vi "ExpressVIElapsedTime.vi"() -> ()   [LabVIEW 2019]
panel:
  in  "stop":bool
  in  "Time Target (s)":dbl=5.0
  out "Boolean":bool
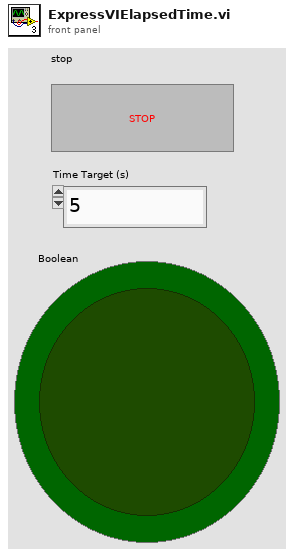
[diagram p1: front panel]
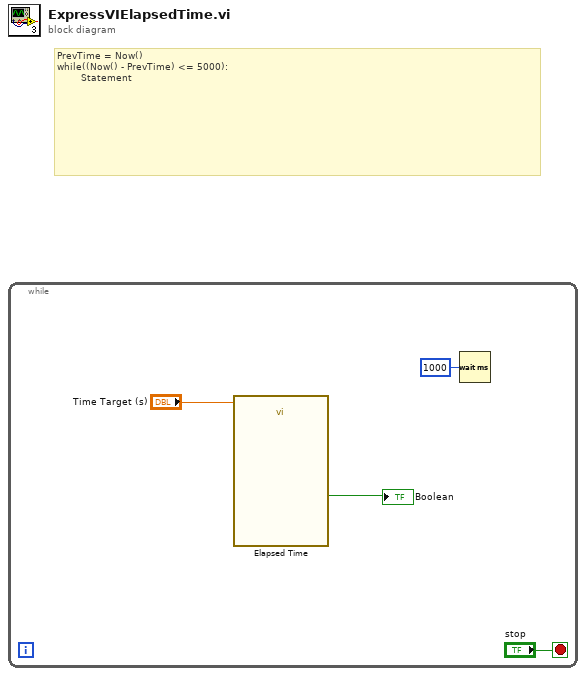
[diagram p0: block diagram]
diagram:
  # "PrevTime = Now()  \nwhile((Now() - PrevTime) <= 5000):\n        Statement"
  n1 = while {
    stop <- "stop" stop-if-true
    n2 = call "Elapsed Time"("Time Target (s)"="Time Target (s)") -> ("Time has Elapsed"=→"Boolean":bool)  [unwired: 11 in, 7 out]
    n3 = Wait (ms)(milliseconds to wait=u32 1000) -> ()  [unwired: 1 out]
  }
